vi "Generate UUID V4 (Random).vi"(8 "error in (no error)":errorcluster) -> (0 "error out":errorcluster, 2 "UUID":string)   [LabVIEW 2015]
uses:
  UUID/Variants.ctl
  UUID/UUID.lvclass
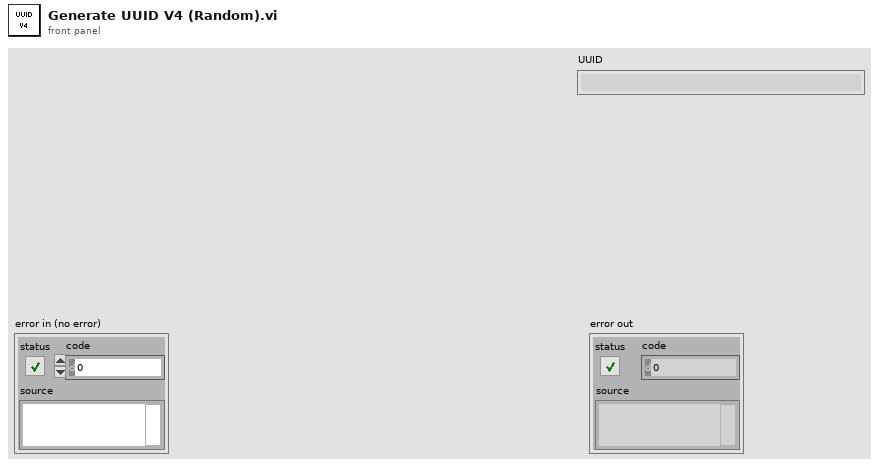
[diagram p1: front panel]
types:
  T1 = typedef "UUID.lvclass/Variants.ctl" = enum16{"NCS", "RFC", "Microsoft"}
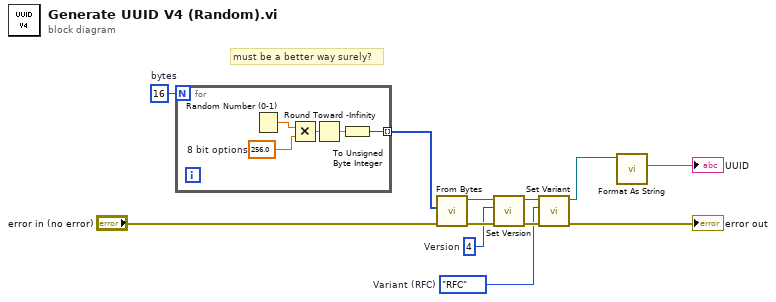
[diagram p0: block diagram]
diagram:
  w1 = Variants."RFC"  # Variant (RFC)
  w2 = u8 4  # Version
  w4 = 16  # bytes
  # "must be a better way surely?"
  n1 = for {
    N: w4 -> [_]
    tunnel: [w13] -> w3 mode=indexing
    w16 = 256.0  # 8 bit options
    n2 = Random Number (0-1)() -> (number: 0 to 1=w17:dbl)
    n3 = Multiply(x=w17, y=w16) -> (x*y=w14:dbl)
    n4 = Round Toward -Infinity(1:w14) -> (0:w15:dbl)
    n5 = To Unsigned Byte Integer(number=w15) -> (unsigned 8bit integer=w13:u8)
  }
  n6 = call "From Bytes.vi"("error in (no error)"="error in (no error)", "Bytes"=w3) -> ("error out"=w6:errorcluster, "UUID out"=w9:refnum<class "UUID.lvclass">)  [unwired: 8 in]
  n7 = call "Set Version.vi"("error in (no error)"=w6, "Version"=w2, "UUID in"=w9) -> ("error out"=w7:errorcluster, "UUID out"=w10:refnum<class "UUID.lvclass">)  [unwired: 7 in]
  n8 = call "Set Variant.vi"("error in (no error)"=w7, "Variant (RFC)"=w1, "UUID in"=w10) -> ("error out"=→"error out":errorcluster, "UUID out"=w12:refnum<class "UUID.lvclass">)  [unwired: 7 in]
  n9 = call "Format As String.vi"("UUID.lvclass"=w12) -> ("String"=→"UUID":string)  [unwired: 10 in]
